vi "FPGA Main.vi"() -> ()   [LabVIEW 2021]
uses:
  <vilib>/Platform/TimedLoop/XDataNode/timing_clust.ctl
  <vilib>/Platform/TimedLoop/XDataNode/nitl_modes.ctl
  <vilib>/Platform/TimedLoop/XDataNode/wakeup.ctl
  <vilib>/rvi/Emulation/niFpgaGetClockAttributes.vi
  <vilib>/rvi/Emulation/niFpgaSctlEmulationGetInTimedLoop.vi
  <vilib>/rvi/Emulation/niFpgaEmulationReportErrorSimple.vi
  <vilib>/rvi/eio/common/nirviEmuTemplateMethod_errors.vi
  <vilib>/rvi/Emulation/niFpgaCriticalErrorInLSC.vi
  <vilib>/eio/EIONode/EIONode.xnode
  <vilib>/platform/TimedLoop/XDataNode/XDataNode.xnode
  <vilib>/Platform/TimedLoop/XDataNode/XDNodeRunTimeDep.lvlib
panel:
  out "loop 1":i32
  in  "Count(mSec)":u32
  out "Led3i":bool
  out "Pause Led2i":bool
  out "Led1i":bool
  out "Led0i":bool
  in  "Pause":bool
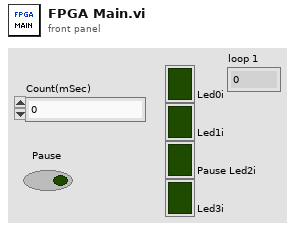
[diagram p1: front panel]
types:
  T1 = typedef "XDNodeRunTimeDep.lvlib/timing_clust.ctl" = cluster{"Expected End [f-1]":u64, "Actual End [f-1]":u64, "Finished Late? [f-1]":bool, "Expected End [i-1]":u64, "Actual End [i-1]":u64, "Finished Late? [i-1]":bool, "Expected Start [i]":u64, "Actual Start [i]":u64, "Expected Start [f]":u64, "Actual Start [f]":u64, "Source Name":string, "Structure Name":string, "Period":i64, "Deadline":i64, "Offset":i64, "Start":i64, "Priority":i32, "Timeout":i32, "Mode":T2, "Wakeup Reason":T3, "Error":errorcluster, "Source Type":string, "Secondary Source Type":string, "Global End Time":u64, "Global Start Time":u64, "Frame Duration":u64, "Iteration Duration":u64, "Assigned CPU":i32, "I/O Scan Engine Mode":u32}
  T2 = typedef "XDNodeRunTimeDep.lvlib/nitl_modes.ctl" = enum32{"No Change", "Process missed periods, maintain original phase", "Discard missed periods, maintain original phase", "Process missed periods, ignore original phase", "Discard missed periods, ignore original phase"}
  T3 = typedef "XDNodeRunTimeDep.lvlib/wakeup.ctl" = enum32{"Normal", "Aborted", "Asynchronous wakeup", "Timing source error", "Timed loop error", "Timeout"}
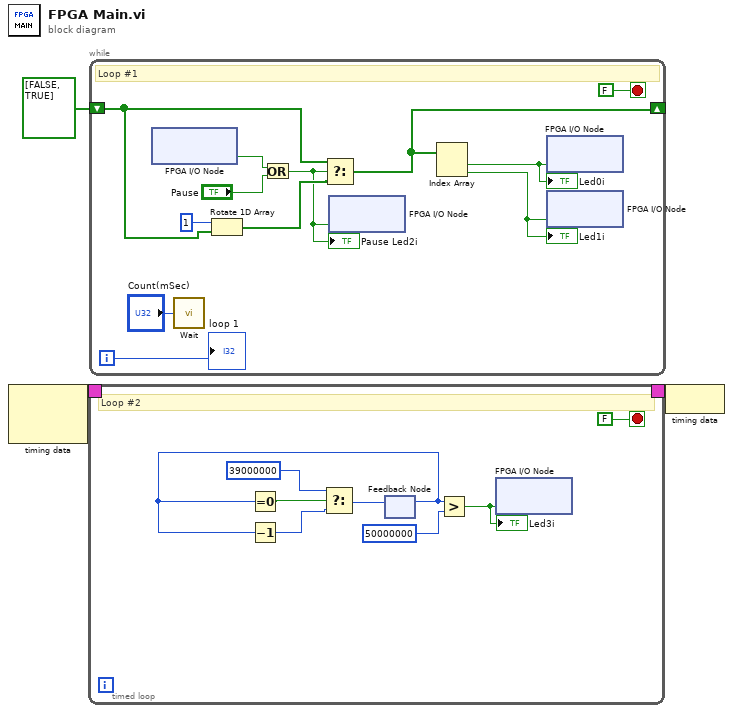
[diagram p0: block diagram]
diagram:
  n1 = node-c288() -> (w2:T1)  [unwired: 2 in]
  n2 = timed-loop {
    timing: w2 -> [_]
    timing-out: [_] -> w1
    stop <- FALSE stop-if-true
    # "Loop #2"
    n3 = feedback #1() -> (w5:u32)  [unwired: 1 in]
    n4 = Equal To 0?(x=w5) -> (x = 0?=w7:bool)
    n5 = Decrement(x=w5) -> (x-1=w6:u32)
    n6 = Select(t=u32 39000000, s=w7, f=w6) -> (s? t:f=w10:u32)
    n7 = feedback-in #1(w10) -> ()
    n8 = Greater?(x=w5, y=u32 50000000) -> (0:w8:bool)
    "Led3i" <- w8
    n9 = xnode "FPGA I/O Node"("LED3"=w8) -> ()  [unwired: 1 in, 1 out]
  }
  n10 = while {
    shift-right: [w18] -> _
    shift-left: bool[] [FALSE, TRUE] -> [w19]
    i -> [w14]
    stop <- FALSE stop-if-true
    # "Loop #1"
    n11 = xnode "FPGA I/O Node"() -> ("Button0"=w25:bool)  [unwired: 1 in, 1 out]
    n12 = call "Wait"("Count(mSec)"="Count(mSec)") -> ()  [unwired: 1 out]
    n13 = Rotate 1D Array(1:w19, 2:1 ("n")) -> (0:w20:bool[])
    n14 = Or(x=w25, y="Pause") -> (x .or. y?=w15:bool)
    "Pause Led2i" <- w15
    n15 = Select(t=w19, s=w15, f=w20) -> (s? t:f=w18:bool[])
    n16 = xnode "FPGA I/O Node"("LED2"=w15) -> ()  [unwired: 1 in, 1 out]
    n17 = Index Array(array=w18) -> (element #1=w17:bool, element #2=w16:bool)  [unwired: 2 in]
    "Led0i" <- w17
    "Led1i" <- w16
    n18 = xnode "FPGA I/O Node"("LED0"=w17) -> ()  [unwired: 1 in, 1 out]
    n19 = xnode "FPGA I/O Node"("LED1"=w16) -> ()  [unwired: 1 in, 1 out]
    "loop 1" <- w14
  }
  n20 = node-c288(w1) -> ()
